vi "Set Class VIs as Inline.vi"(8 "error in (no error)":errorcluster, 11 "class ref":refnum<vi>) -> (0 "error out":errorcluster, 3 "class vi refs":refnum<vi>[](array[refnum]))   [LabVIEW 2017, in "Build Automation.lvlib"]
uses:
  Build Automation.lvlib
  VI Options.ctl
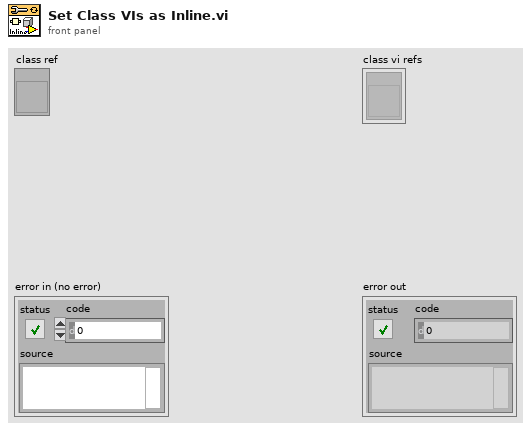
[diagram p1: front panel]
types:
  T1 = typedef "Build Automation.lvlib/VI Options.ctl" = cluster{"Inline":bool, "Is Reentrant":bool, "Reentrancy Type":enum16{"Share clones between instances", "Preallocate clone for each instance"}, "Enable Debugging":bool}
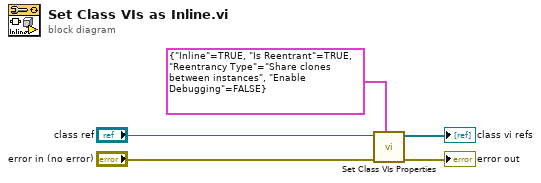
[diagram p0: block diagram]
diagram:
  n1 = call "Set Class VIs Properties.vi"("VI Options"=T1 {"Inline"=TRUE, "Is Reentrant"=TRUE, "Reentrancy Type"=enum."Share clones between instances", "Enable Debugging"=FALSE}, "error in (no error)"="error in (no error)", "class ref"="class ref") -> ("error out"=→"error out":errorcluster, "class vi refs"=→"class vi refs":refnum<vi>[])  [unwired: 7 in]
